vi "Monitor.vi"(8 "error In":errorcluster {"code" format="%.0x"}) -> (0 "error Out":errorcluster, 2 "Wiek 2":i32, 3 "imie 2":string)   [LabVIEW 2024]
panel:
  out "String":string
  in  "Wiek":i32
  in  "Imie":string
  in  "OK":bool
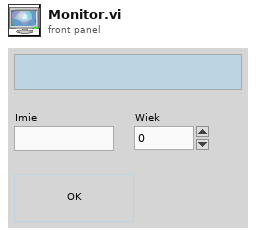
[diagram p1: front panel]
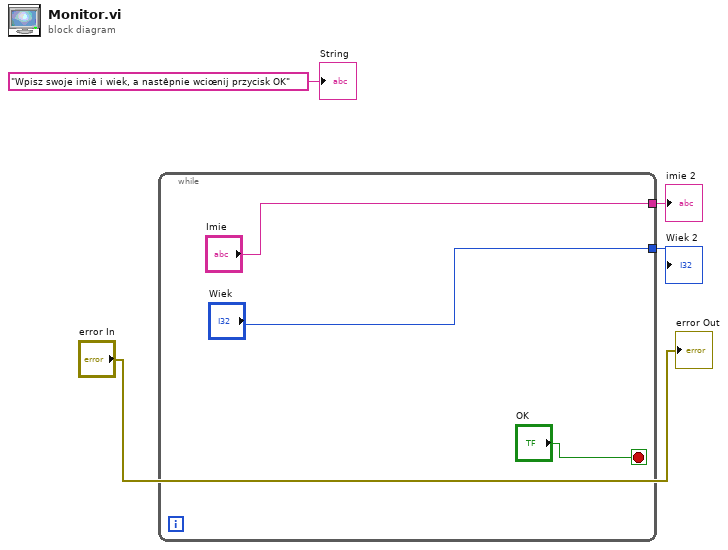
[diagram p0: block diagram]
diagram:
  n1 = while {
    tunnel: ["Imie"] -> w3
    tunnel: ["Wiek"] -> w2
    stop <- "OK" stop-if-true
  }
  "imie 2" <- w3
  "Wiek 2" <- w2
  "error Out" <- "error In"
  "String" <- "Wpisz swoje imiê i wiek, a nastêpnie wciœnij przycisk OK" ("String")
